vi "CSM - Filter Global Log.vi"   [LabVIEW 2020, in "Communicable State Machine.lvlib"]
uses:
  Communicable State Machine.lvlib
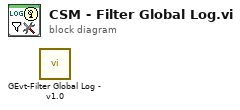
[diagram p0: block diagram]
diagram:
  n1 = call "GEvt-Filter Global Log - v1.0.vi"() -> ()  [unwired: 10 in, 2 out]
